vi "UI--Settings by Name.vi"(8 "error in":errorcluster, 9 "Settings":T1, 10 "Names":string[](array[string]), 11 "Selector in":refnum<class "Selector.lvclass">) -> (0 "error out":errorcluster, 3 "Selector out":refnum<class "Selector.lvclass">)   [LabVIEW 2019, in "Selector.lvclass"]
uses:
  Selector.lvclass
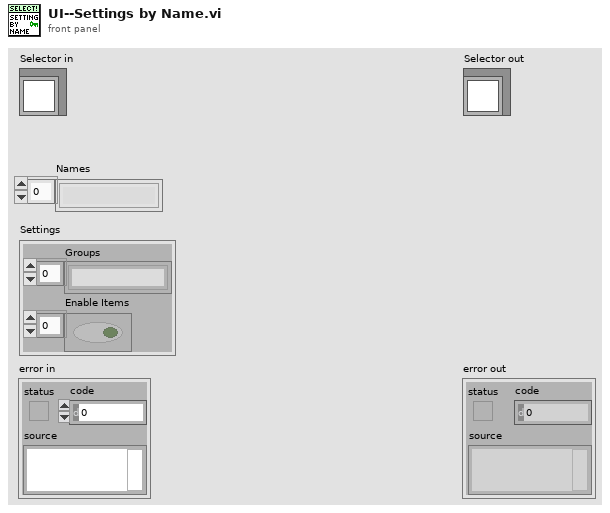
[diagram p1: front panel]
types:
  T1 = cluster{"Groups":string[], "Enable Items":bool[]}
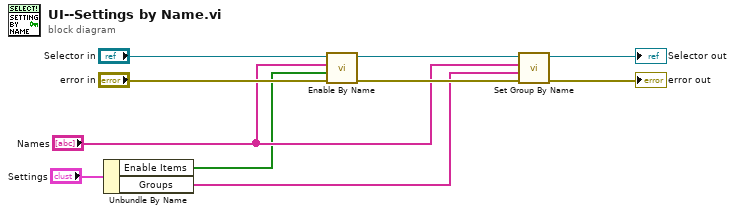
[diagram p0: block diagram]
diagram:
  n1 = Unbundle By Name("Settings") -> ("Enable Items"=w2:bool[], "Groups"=w1:string[])
  n2 = call-dynamic "Enable By Name.vi"("error in (no error)"="error in", "Enable Items"=w2, "Names"="Names", "Selector in"="Selector in") -> ("error out"=w8:errorcluster, "Selector out"=w7:refnum<class "Selector.lvclass">)  [unwired: 6 in]
  n3 = call "Set Group By Name.vi"("error in (no error)"=w8, "Groups"=w1, "Names"="Names", "Selector in"=w7) -> ("error out"=→"error out":errorcluster, "Selector out"=→"Selector out":refnum<class "Selector.lvclass">)  [unwired: 6 in]
